vi "Simple SPIKE IDE.vi"() -> ()   [LabVIEW 2020]
panel:
  in  "New File":bool
  in  "Py Files":i32(listbox)
  in  "Python Files":path
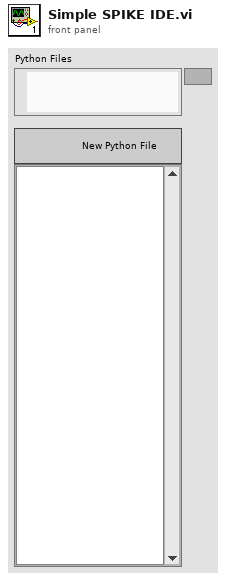
[diagram p1: front panel]
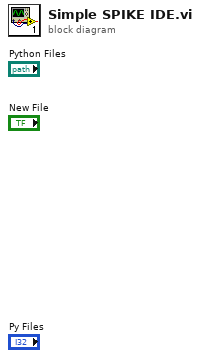
[diagram p0: block diagram]
diagram:
